vi "Load Front Panel control values from cfg file.vi"(6 "Val(Sgnl)? (False)":bool, 7 "error in":errorcluster, 8 "Enable?":bool, 9 "GUI":T1, 10 "VI reference":refnum<vi>) -> (0 "error out":errorcluster, 1 "Controls Changed?":bool, 3 "VI reference out":refnum<vi>)   [LabVIEW 2013]
doc: "This .vi retrieves the flattened control values from file. If a control is missing/changed, That control is not changed."
uses:
  HHMI - Config file functional global mode enum.ctl
  User interface config file selector enum.ctl
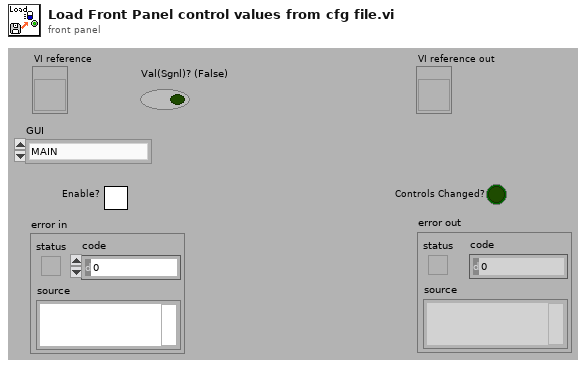
[diagram p1: front panel]
types:
  T1 = typedef "User interface config file selector enum.ctl" = enum16{"MAIN"}
  T2 = typedef "HHMI - Config file functional global mode enum.ctl" = enum16{"Set Filepath", "Read file", "Rewrite file"}
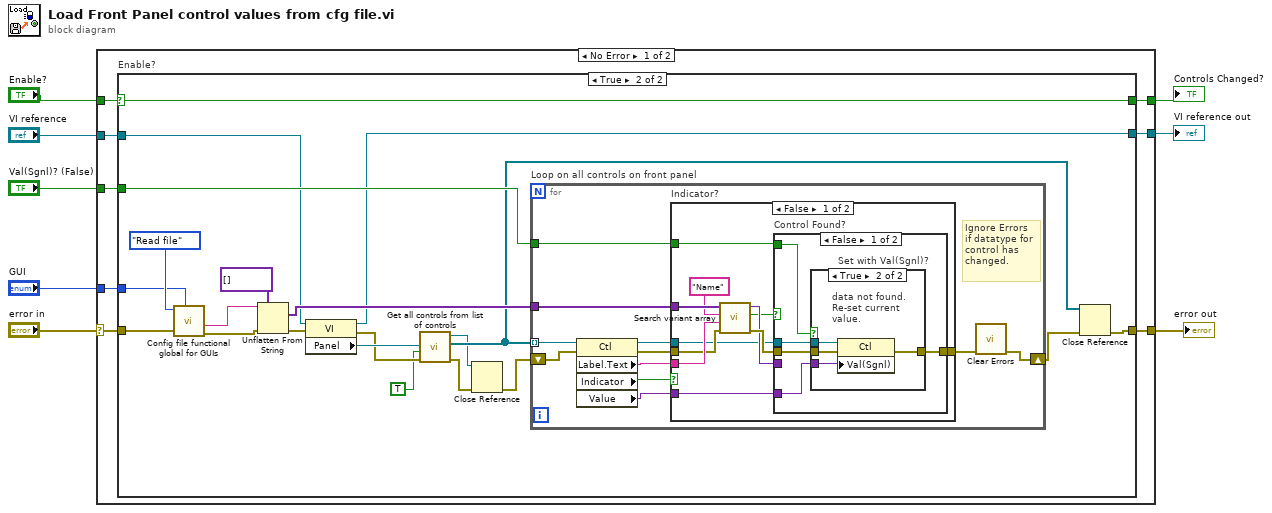
[diagram p0: block diagram]
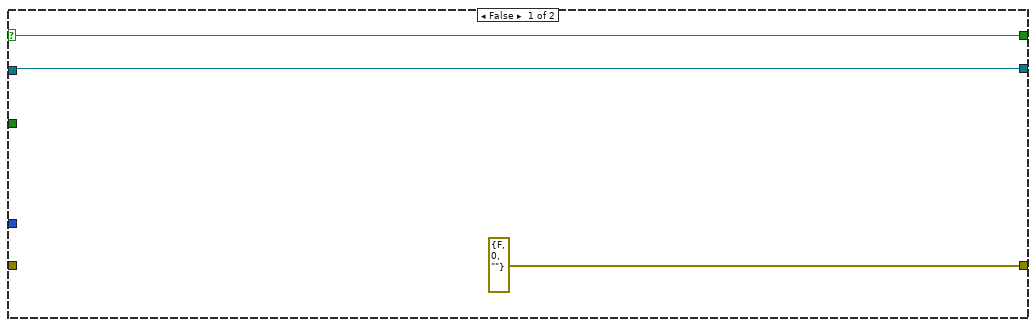
[diagram p2: hidden frame]
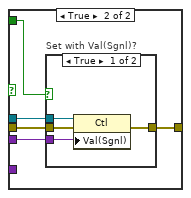
[diagram p4: hidden frame]
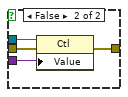
[diagram p5: hidden frame]
diagram:
  n1 = case shown="No Error" "error in" {
    selector: "error in" -> [w11 w89]
    tunnel: [w16 w89] -> w8
    tunnel: "VI reference" -> [w15 w88]
    tunnel: [w14 w88] -> w6
    tunnel: "Enable?" -> [w13 w87]
    tunnel: [w12 w87] -> w4
    tunnel: "GUI" -> [w10 _]
    tunnel: "Val(Sgnl)? (False)" -> [w9 _]
    frame No Error {
      n2 = case "Enable?" shown="True" w13 {
        selector: w13 -> [w18 w38]
        tunnel: [errorcluster {"status"=FALSE, "code"=0, "source"=""} ("error out") w23] -> w16
        tunnel: w15 -> [w19 w28]
        tunnel: [w19 w29] -> w14
        tunnel: [w18 w38] -> w12
        tunnel: w11 -> [_ w36]
        tunnel: w10 -> [_ w32]
        tunnel: w9 -> [_ w40]
        frame False {
        }
        frame True {
          n3 = call "Config file functional global for GUIs.vi"("GUI elements"=w32, "error in"=w36, "Mode"=HHMI_-_Config_file_functional_global_mode_enum."Read file") -> ("error out"=w35:errorcluster, "text read"=w34:string)  [unwired: 2 in, 5 out]
          n4 = Unflatten From String(type=variant[] [], binary string=w34, error in (no error)=w35) -> (value=w39:variant[], error out=w31:errorcluster)  [unwired: 3 out]
          n5 = property class="VI"(reference=w28, error in=w31) -> (reference out=w29:refnum<vi>, error out=w25:errorcluster, "Panel"=w26:refnum<vi>)
          n6 = call "Get all controls from list of controls.vi"("error in"=w25, "Exclude tabs?"=TRUE, "VI Panel"=w26) -> ("error out"=w21:errorcluster, "All Controls (except/incl tabs) []"=w27:refnum<vi>[], "VI Panel refout"=w22:refnum<vi>)  [unwired: 6 out]
          n7 = Close Reference(reference=w22, error in (no error)=w21) -> (error out=w20:errorcluster)
          n8 = for "Loop on all controls on front panel" {
            tunnel: w27 -> [w42] mode=indexing
            shift-right: [w50] -> w30
            shift-left: w20 -> [w49]
            tunnel: w39 -> [w51]
            tunnel: w40 -> [w44]
            # "Ignore Errors\nif datatype for\ncontrol has \nchanged."
            n9 = property class="Ctl"(reference=w42, error in=w49) -> (reference out=w46:refnum<vi>, error out=w47:errorcluster, "Label.Text"=w48:string, "Indicator"=w43:bool, "Value"=w41:variant)
            n10 = case "Indicator?" shown="False" w43 {
              tunnel: w51 -> [w62 _]
              tunnel: w48 -> [w57 _]
              tunnel: w47 -> [w56 w86]
              tunnel: w46 -> [w55 _]
              tunnel: [w54 w86] -> w45
              tunnel: w44 -> [w53 _]
              tunnel: w41 -> [w52 _]
              frame False {
                n11 = call "Search variant array.vi"("error in"=w56, "Text to match"=w57, "Tag name"="Name", "Array"=w62) -> ("error out"=w60:errorcluster, "Found?"=w58:bool, "Variant"=w59:variant)  [unwired: 5 out]
                n12 = case "Control Found?" shown="False" w58 {
                  tunnel: w60 -> [w66 w77]
                  tunnel: [w65 w76] -> w54
                  tunnel: w59 -> [_ w74]
                  tunnel: w55 -> [w67 w75]
                  tunnel: w53 -> [w64 w73]
                  tunnel: w52 -> [w63 _]
                  frame False {
                    n13 = case "Set with Val(Sgnl)?" shown="True" w64 {
                      tunnel: w67 -> [_ w72]
                      tunnel: w66 -> [w68 w71]
                      tunnel: [w68 w70] -> w65
                      tunnel: w63 -> [_ w69]
                      frame False {
                      }
                      frame True {
                        # "data not found.\nRe-set current\nvalue."
                        n14 = property class="Ctl"(reference=w72, error in=w71, "Val(Sgnl)"=w69) -> (error out=w70:errorcluster)  [unwired: 1 out]
                      }
                    }
                  }
                  frame True {
                    n15 = case "Set with Val(Sgnl)?" shown="True" w73 {
                      tunnel: w77 -> [w81 w85]
                      tunnel: [w80 w84] -> w76
                      tunnel: w75 -> [w79 w83]
                      tunnel: w74 -> [w78 w82]
                      frame True {
                        n16 = property class="Ctl"(reference=w79, error in=w81, "Val(Sgnl)"=w78) -> (error out=w80:errorcluster)  [unwired: 1 out]
                      }
                      frame False {
                        n17 = property class="Ctl"(reference=w83, error in=w85, "Value"=w82) -> (error out=w84:errorcluster)  [unwired: 1 out]
                      }
                    }
                  }
                }
              }
              frame True {
                # "Indicator."
              }
            }
            n18 = call <vilib>:"Clear Errors.vi"("error in (no error)"=w45) -> ("error out"=w50:errorcluster)  [unwired: 6 out]
          }
          n19 = Close Reference(reference=w27, error in (no error)=w30) -> (error out=w23:errorcluster)
        }
      }
    }
    frame Error {
    }
  }
  "error out" <- w8
  "VI reference out" <- w6
  "Controls Changed?" <- w4
